vi "filterVelocityPeak.vi"(4 "empty?":bool, 6 "dt":dbl, 7 "x_k|k":T1, 8 "error in (no error)":errorcluster, 9 "vel_y":dbl, 10 "vel_x":dbl, 11 "Vision in":refnum<class "Vision.lvclass">) -> (0 "error out":errorcluster, 1 "vel_y out":dbl, 2 "vel_x out":dbl, 3 "Vision out":refnum<class "Vision.lvclass">)   [LabVIEW 2021, in "Vision.lvclass"]
uses:
  Vision.lvclass
  <vilib>/Analysis/Matrix/Datatypes/RealMatrix.ctl
  <vilib>/Analysis/Matrix/NI_Matrix.lvlib
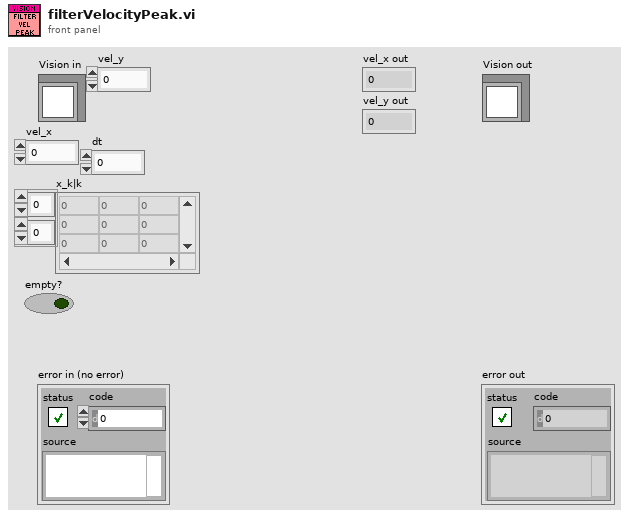
[diagram p1: front panel]
types:
  T1 = typedef "NI_Matrix.lvlib/RealMatrix.ctl" = dbl[][]
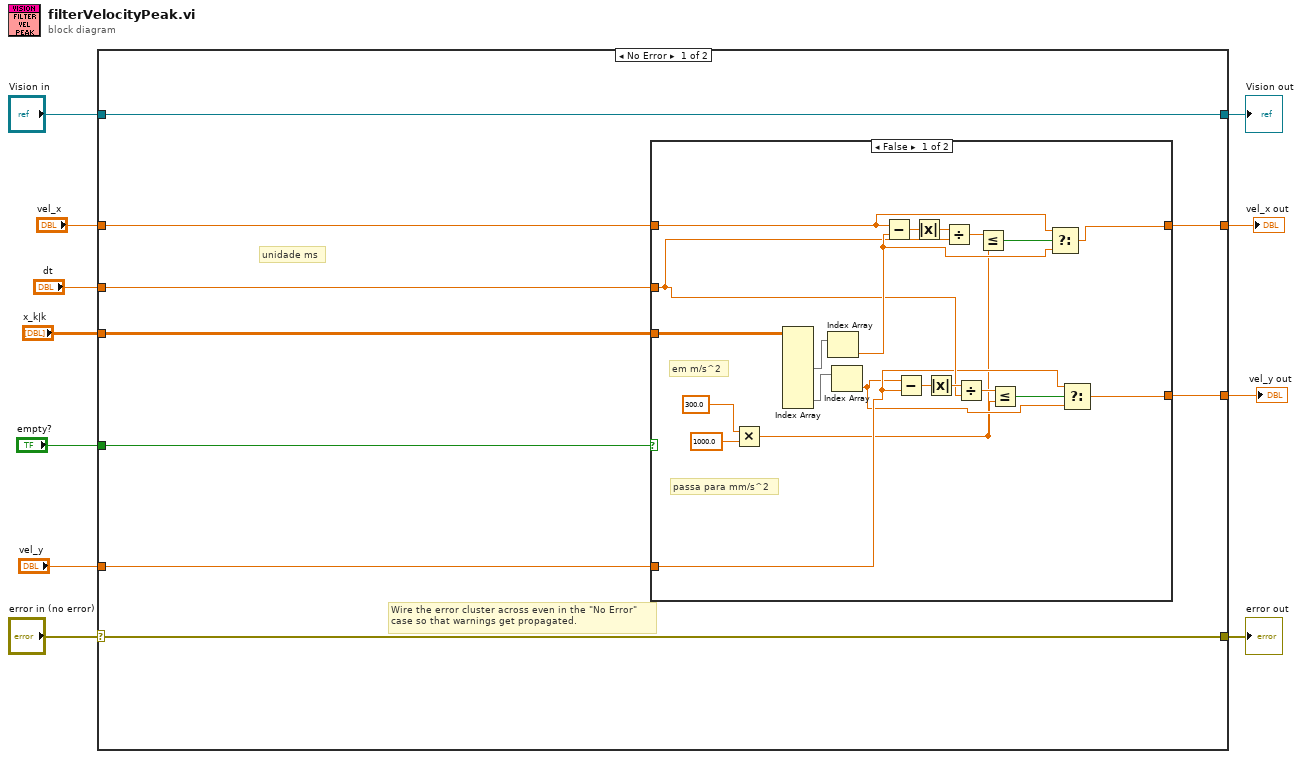
[diagram p0: block diagram]
diagram:
  n1 = case shown="No Error" "error in (no error)" {
    selector: "error in (no error)" -> [w19 w45]
    tunnel: [w19 w45] -> w10
    tunnel: [w20 w44] -> w8
    tunnel: "Vision in" -> [w20 w44]
    tunnel: "vel_x" -> [w18 _]
    tunnel: "vel_y" -> [w17 _]
    tunnel: [w16 _] -> w5
    tunnel: [w15 _] -> w4
    tunnel: "dt" -> [w14 _]
    tunnel: "x_k|k" -> [w13 _]
    tunnel: "empty?" -> [w12 _]
    frame No Error {
      # "unidade ms"
      # "Wire the error cluster across even in the \"No Error\"\ncase so that warnings get propagated."
      n2 = case shown="False" w12 {
        tunnel: w18 -> [w36 w43]
        tunnel: [w34 w43] -> w16
        tunnel: w17 -> [w27 w42]
        tunnel: [w29 w42] -> w15
        tunnel: w14 -> [w28 _]
        tunnel: w13 -> [w22 _]
        frame False {
          # "passa para mm/s^2"
          # "em m/s^2"
          n3 = Multiply(x=300.0, y=1000.0) -> (x*y=w23:dbl)
          n4 = Index Array(array=w22) -> (element #2=w41:dbl[], element #4=w40:dbl[])  [unwired: 8 in, 2 out]
          n5 = Index Array(array=w41) -> (element=w35:dbl)  [unwired: 1 in]
          n6 = Index Array(array=w40) -> (element=w26:dbl)  [unwired: 1 in]
          n7 = Subtract(x=w36, y=w35) -> (x-y=w39:dbl)
          n8 = Subtract(x=w26, y=w27) -> (x-y=w33:dbl)
          n9 = Absolute Value(x=w39) -> (abs(x)=w38:dbl)
          n10 = Absolute Value(x=w33) -> (abs(x)=w32:dbl)
          n11 = Divide(x=w38, y=w28) -> (x/y=w21:dbl)
          n12 = Divide(x=w32, y=w28) -> (x/y=w31:dbl)
          n13 = Less Or Equal?(x=w21, y=w23) -> (x <= y?=w37:bool)
          n14 = Less Or Equal?(x=w31, y=w23) -> (x <= y?=w30:bool)
          n15 = Select(t=w36, s=w37, f=w35) -> (s? t:f=w34:dbl)
          n16 = Select(t=w27, s=w30, f=w26) -> (s? t:f=w29:dbl)
        }
        frame True {
          # "Bola com esse id não existe mais"
        }
      }
    }
    frame Error {
    }
  }
  "error out" <- w10
  "Vision out" <- w8
  "vel_x out" <- w5
  "vel_y out" <- w4
